vi "Create.vi"(6 "Use Hardware Acceleration (Default: F)":bool, 7 "Fourcc":T2, 8 "error in (no error)":errorcluster, 9 "Frames Per Second":dbl, 10 "Image Size":T1, 11 "Path":path) -> (0 "error out":errorcluster, 3 "Writer (Greyscale)":refnum<class "Writer (Greyscale).lvclass">)   [LabVIEW 2020, in "video_io.lvlib" / "Writer (Greyscale).lvclass"]
uses:
  Writer (Greyscale).lvclass
  FourCC.ctl
  common/Image Size (Integer).ctl
  Writer (Greyscale).lvclass/Writer (Greyscale).ctl
  <vilib>/Utility/error.llb/Error Cluster From Error Code.vi
  video_io.lvlib
  common/common.lvlib
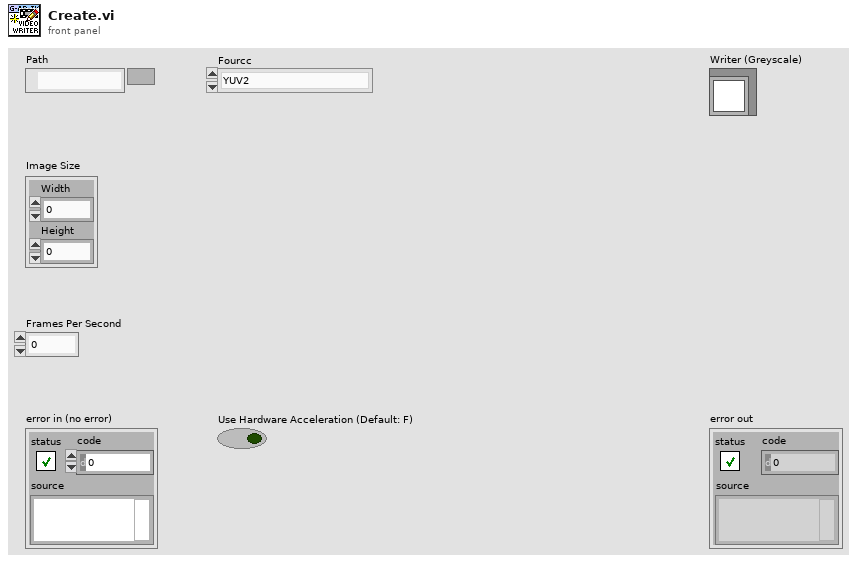
[diagram p1: front panel]
types:
  T1 = typedef "common.lvlib/Image Size (Integer).ctl" = cluster{"Width":u16, "Height":u16}
  T2 = typedef "video_io.lvlib/FourCC.ctl" = enum16{"YUV2", "2VUY", "YUVS", "RGBA", "YUV4", "JPEG", "MJPA", "AVDJ", "DMB1", "MP4V", "DIVX", "XVID", "3IV2", "S263", "AVC1", "AI5P", "AI5Q", "AI52", "AI53", "AI55", "AI56", "AI1P", "AI1Q", "AI12", "AI13", "AI15", "AI16", "M1V1", "MPEG", "M2V1", "HDV1", "HDV2", "HDV3", "HDV4", "HDV5", "HDV6", "HDV7", "HDV8", "HDV9", "HDVA", "MX5N", "MX5P", "MX4N", "MX4P", "MX3N", "MX3P", "XD54", "XD55", "XD59", "XD5A", "XD5B", "XD5C", "XD5D", "XD5E", "XD5F", "XDV1", "XDV2", "XDV3", "XDV4", "XDV5", "XDV6", "XDV7", "XDV8", "XDV9", "XDVA", "XDVB", "XDVC", "XDVD", "XDVE", "XDVF", "XDHD", "XDH2", "AVMP", "MJP2", "TIFF", "DRAC", "3IVD", "L555", "L565", "B565", "24BG", "BGRA", "ABGR", "B16G", "B48R", "BXBG", "BXRG", "BXYV", "NO16", "DVOO", "R420", "R411", "WRAW", "AV1X", "AVUP"}
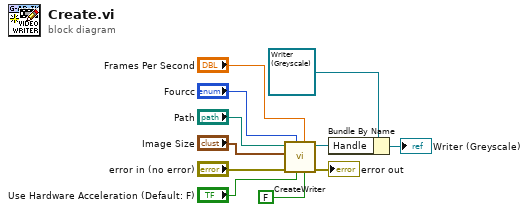
[diagram p0: block diagram]
diagram:
  n1 = call "CreateWriter.vi"("Is Colour"=FALSE, "Frames Per Second"="Frames Per Second", "Use HW"="Use Hardware Acceleration (Default: F)", "Fourcc"="Fourcc", "error in (no error)"="error in (no error)", "Image Size"="Image Size", "Path"="Path") -> ("error out"=→"error out":errorcluster, "Data Value Reference out"=w4:refnum<data-value>)  [unwired: 3 in]
  n2 = Bundle By Name(cluster=refnum<class "Writer (Greyscale).lvclass"> refnum ("video_io.lvlib:Writer (ARGB).lvclass"), "Handle"=w4) -> (→"Writer (Greyscale)":refnum<class "Writer (Greyscale).lvclass">)
